vi "Check Status.vi"(8 "error in (no error)":errorcluster, 11 "Lakeshore Gaussmeter in":refnum<class "Lakeshore Gaussmeter.lvclass">) -> (0 "error out":errorcluster, 1 "Status":string, 2 "Ready?":bool, 3 "Lakeshore Gaussmeter out":refnum<class "Lakeshore Gaussmeter.lvclass">)   [LabVIEW 2017, in "Lakeshore Gaussmeter.lvclass"]
doc: "(Dynamic) Check if the instrument is powered on and update its member fields with the instrument's current status. Optionally return a text status message."
uses:
  Lakeshore Gaussmeter.lvclass
  Lakeshore Gaussmeter.lvclass/Lakeshore Gaussmeter.ctl
  Utility Classes/Scannable/Scannable.lvclass
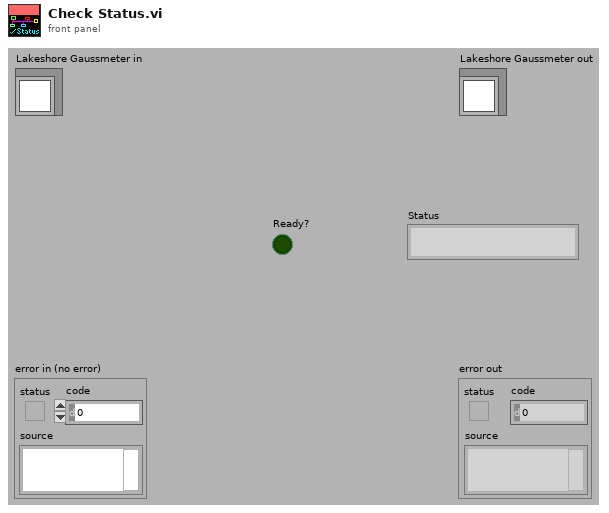
[diagram p1: front panel]
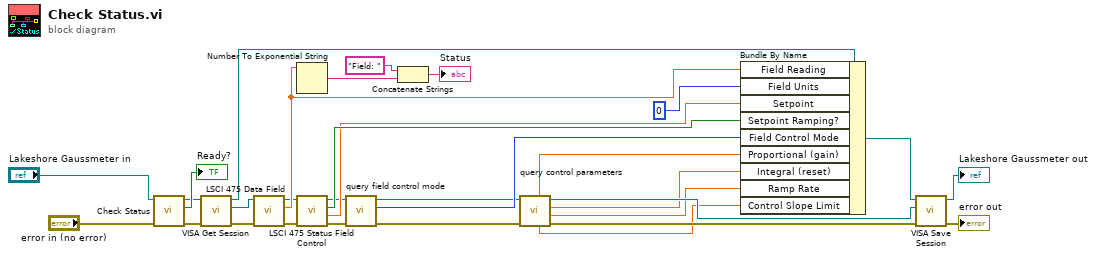
[diagram p0: block diagram]
diagram:
  n1 = call-parent "Check Status.vi"("error in (no error)"="error in (no error)", "Instrument in"="Lakeshore Gaussmeter in") -> ("error out"=w18:errorcluster, "Ready?"=→"Ready?":bool, "Instrument out"=w28:refnum<class "Lakeshore Gaussmeter.lvclass">)  [unwired: 6 in, 1 out]
  n2 = call-dynamic "VISA Get Session.vi"("error in (no error)"=w18, "Instrument.lvclass in"=w28) -> ("error out"=w19:errorcluster, "VISA Resource Name"=w20:refnum<visa-resource-name>, "Instrument.lvclass out"=w27:refnum<class "Lakeshore Gaussmeter.lvclass">)  [unwired: 7 out]
  n3 = call "LSCI 475 Data Field.vi"("error in (no error)"=w19, "VISA session"=w20) -> ("error out"=w14:errorcluster, "Field Reading"=w17:dbl, "dup VISA session"=w15:refnum<visa-resource-name>)  [unwired: 7 in]
  n4 = Number To Exponential String(number=w17) -> (E-format string=w16:string)  [unwired: 3 in]
  n5 = call "LSCI 475 Status Field Control.vi"("error in (no error)"=w14, "VISA session"=w15) -> ("error out"=w10:errorcluster, "Present Setpoint"=w12:dbl, "Setpoint Ramping?"=w13:bool, "dup VISA session"=w11:refnum<visa-resource-name>)  [unwired: 6 in]
  n6 = call "query field control mode.vi"("error in (no error)"=w10, "VISA session"=w11) -> ("error out"=w6:errorcluster, "Field Control Mode (0: Off)"=w9:u16, "dup VISA session"=w8:refnum<visa-resource-name>)  [unwired: 7 in]
  n7 = Concatenate Strings("Field: ", w16) -> (→"Status":string)
  n8 = call "query control parameters.vi"("error in (no error)"=w6, "VISA session"=w8) -> ("error out"=w5:errorcluster, "Ramp Rate"=w2:dbl, "Integral (reset)"=w3:dbl, "dup VISA session"=w7:refnum<visa-resource-name>, "Control Slope Limit"=w1:dbl, "Proportional (gain)"=w4:dbl)  [unwired: 4 in]
  n9 = Bundle By Name(cluster=w27, "Field Reading"=w17, "Field Units"=u16 0 ("Field Units (0: Gauss)"), "Setpoint"=w12, "Setpoint Ramping?"=w13, "Field Control Mode"=w9, "Proportional (gain)"=w4, "Integral (reset)"=w3, "Ramp Rate"=w2, "Control Slope Limit"=w1) -> (w26:refnum<class "Lakeshore Gaussmeter.lvclass">)
  n10 = call-dynamic "VISA Save Session.vi"("error in (no error)"=w5, "VISA Resource Name"=w7, "Instrument.lvclass in"=w26) -> ("error out"=→"error out":errorcluster, "Instrument.lvclass out"=→"Lakeshore Gaussmeter out":refnum<class "Lakeshore Gaussmeter.lvclass">)  [unwired: 7 out]
